vi "instrumentos remotos.vi"() -> ()   [LabVIEW 2020]
uses:
  <vilib>/httpClient/LabVIEWHTTPClient.lvlib
panel:
  out "temperatura":dbl
  out "lateral":bool
  out "frontal":bool
  out "Fecha":string
  out "Humedad":dbl
  out "error out":errorcluster
  out "String":string
  out "String 2":string
  in  "stop":bool
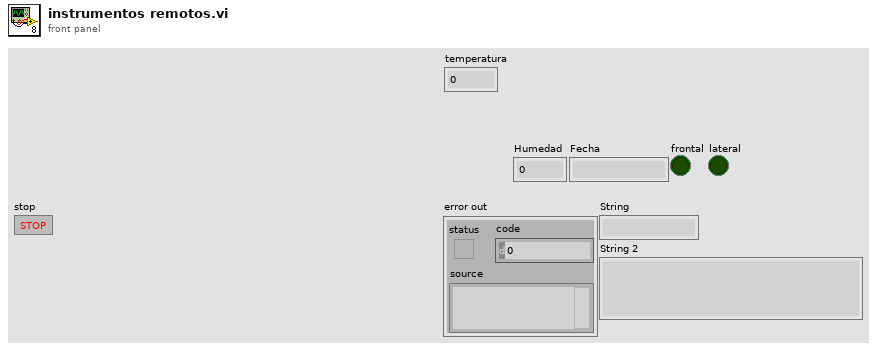
[diagram p1: front panel]
types:
  T1 = cluster{"Humedad":dbl, "Fecha":string, "frontal":bool, "temperature":dbl, "lateral":bool}
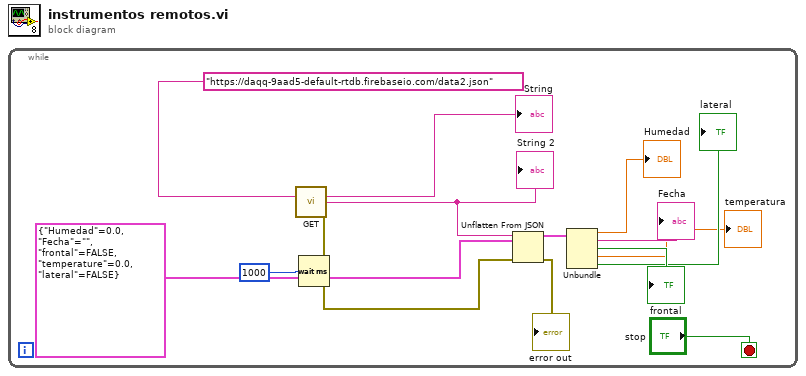
[diagram p0: block diagram]
diagram:
  n1 = while {
    stop <- "stop" stop-if-true
    n2 = call <vilib>:"GET.vi"("url"="https://daqq-9aad5-default-rtdb.firebaseio.com/data2.json") -> ("headers"=→"String":string, "body"=w8:string, "error out"=w10:errorcluster)  [unwired: 11 in, 1 out]
    "String 2" <- w8
    n3 = Wait (ms)(milliseconds to wait=1000) -> ()  [unwired: 1 out]
    n4 = Unflatten From JSON(JSON string=w8, type and defaults=T1 {"Humedad"=0.0, "Fecha"="", "frontal"=FALSE, "temperature"=0.0, "lateral"=FALSE}, error in (no error)=w10) -> (value=w6:T1, error out=→"error out":errorcluster)  [unwired: 4 in]
    n5 = Unbundle(w6) -> ("Humedad"=→"Humedad":dbl, "Fecha"=→"Fecha":string, "frontal"=→"frontal":bool, "temperature"=→"temperatura":dbl, "lateral"=→"lateral":bool)
  }
